vi "Channels data blend.vi"(8 "error in (no error)":errorcluster, 10 "GREEN":T1, 11 "RED":T1) -> (0 "error out":errorcluster, 3 "Image Out":T1)   [LabVIEW 2020]
uses:
  <vilib>/vision/Image Controls.llb/IMAQ Image.ctl
  <vilib>/vision/NI_Vision_Development_Module.lvlib
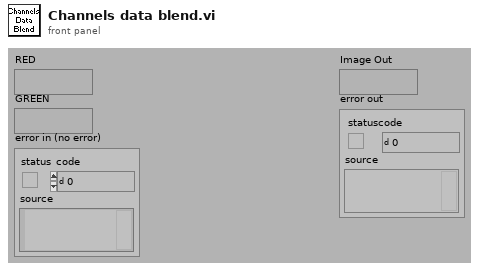
[diagram p1: front panel]
types:
  T1 = typedef "IMAQ Image.ctl" = refnum<image>
  T2 = typedef "Image Type" = u32
  T3 = cluster{"Red or Hue value":u8, "Green or Sat value":u8, "Blue or Luma or Val or Inten value":u8}
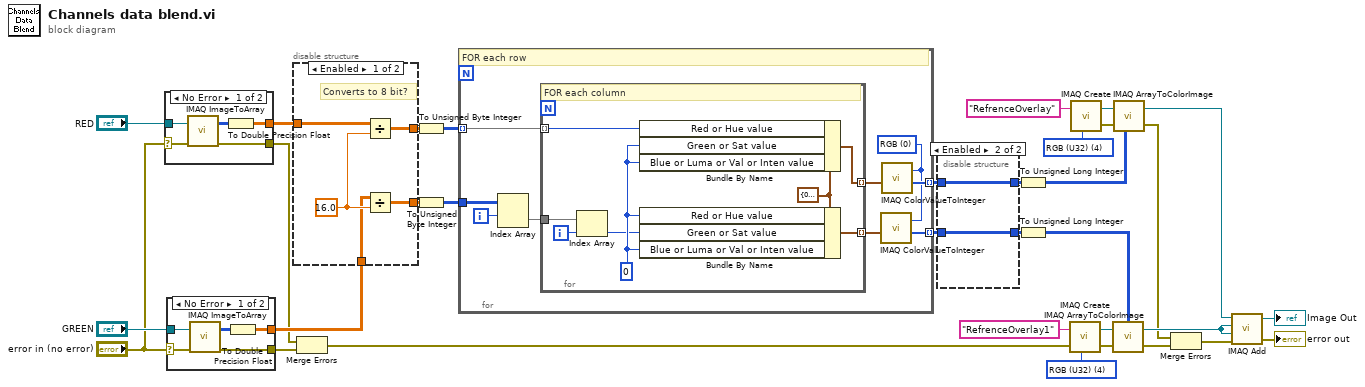
[diagram p0: block diagram]
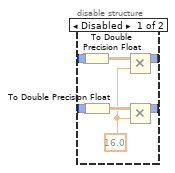
[diagram p2: hidden frame]
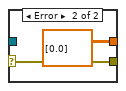
[diagram p4: hidden frame]
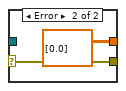
[diagram p5: hidden frame]
diagram:
  w28 = T2 4 items=["Grayscale (U8)", "Grayscale (I16)", "Grayscale (SGL)", "Complex (CSG)", "RGB (U32)", "HSL (U32)", "RGB (U64)", "Grayscale (U16)"] ("Image Type")
  w33 = T2 4 items=["Grayscale (U8)", "Grayscale (I16)", "Grayscale (SGL)", "Complex (CSG)", "RGB (U32)", "HSL (U32)", "RGB (U64)", "Grayscale (U16)"] ("Image Type")
  n1 = case shown="No Error" "error in (no error)" {
    selector: "error in (no error)" -> [w36 w39]
    tunnel: [w34 dbl[][] [[0.0]] ("Image Pixels (I16)")] -> w11
    tunnel: "RED" -> [w38 _]
    tunnel: [w37 w39] -> w9
    frame No Error {
      n2 = call "IMAQ ImageToArray"("error in (no error)"=w36, "Image"=w38) -> ("error out"=w37:errorcluster, "Image Pixels (I16)"=w35:i16[][])  [unwired: 2 in, 3 out]
      n3 = To Double Precision Float(number=w35) -> (double precision float=w34:dbl[][])
    }
    frame Error {
    }
  }
  n4 = case shown="No Error" "error in (no error)" {
    selector: "error in (no error)" -> [w43 w46]
    tunnel: [w41 dbl[][] [[0.0]] ("Image Pixels (I16)")] -> w13
    tunnel: "GREEN" -> [w45 _]
    tunnel: [w44 w46] -> w7
    frame No Error {
      n5 = call "IMAQ ImageToArray"("error in (no error)"=w43, "Image"=w45) -> ("error out"=w44:errorcluster, "Image Pixels (I16)"=w42:i16[][])  [unwired: 2 in, 3 out]
      n6 = To Double Precision Float(number=w42) -> (double precision float=w41:dbl[][])
    }
    frame Error {
    }
  }
  n7 = disable-structure shown="Enabled" {
    disable-tunnel: [w52 w54] -> w21
    disable-tunnel: [w51 w53] -> w19
    disable-tunnel: w13 -> [w49 w53]
    disable-tunnel: w11 -> [w48 w54]
    frame Enabled {
      w50 = 16.0
      # "Converts to 8 bit?"
      n8 = Divide(x=w48, y=w50) -> (x/y=w52:dbl[][])
      n9 = Divide(x=w49, y=w50) -> (x/y=w51:dbl[][])
    }
    frame Disabled {
    }
  }
  n10 = Merge Errors(w9, w7) -> (w8:errorcluster)
  n11 = To Unsigned Byte Integer(number=w21) -> (unsigned 8bit integer=w20:u8[][])
  n12 = To Unsigned Byte Integer(number=w19) -> (unsigned 8bit integer=w18:u8[][])
  n13 = for {
    tunnel: w20 -> [w63] mode=indexing
    tunnel: w18 -> [w58]
    tunnel: [w59] -> w5 mode=indexing
    tunnel: [w61] -> w2 mode=indexing
    i -> [w56]
    w55 = u16 0 items=["RGB", "HSL", "HSV", "HSI"] ("Color Mode")
    # "FOR each row"
    n14 = Index Array(array=w58, index (row)=w56) -> (element=w57:u8[])  [unwired: 1 in]
    n15 = for {
      tunnel: w63 -> [w71] mode=indexing
      tunnel: w57 -> [w66]
      tunnel: [w69] -> w62 mode=indexing
      tunnel: [w68] -> w60 mode=indexing
      i -> [w65]
      w67 = T3 {"Red or Hue value"=0, "Green or Sat value"=0, "Blue or Luma or Val or Inten value"=0} ("Color Value")
      w70 = u8 0
      # "FOR each column"
      n16 = Index Array(array=w66, index=w65) -> (element=w64:u8)
      n17 = Bundle By Name(cluster=w67, "Red or Hue value"=w71, "Green or Sat value"=w70, "Blue or Luma or Val or Inten value"=w70) -> (w68:T3)
      n18 = Bundle By Name(cluster=w67, "Red or Hue value"=w70, "Green or Sat value"=w64, "Blue or Luma or Val or Inten value"=w70) -> (w69:T3)
    }
    n19 = call "IMAQ ColorValueToInteger"("1D Color value array"=w62, "Color Mode"=w55) -> ("1D U32 array"=w61:u32[])  [unwired: 3 in, 3 out]
    n20 = call "IMAQ ColorValueToInteger"("1D Color value array"=w60, "Color Mode"=w55) -> ("1D U32 array"=w59:u32[])  [unwired: 3 in, 3 out]
  }
  n21 = disable-structure shown="Enabled" {
    disable-tunnel: [w78 w80] -> w6
    disable-tunnel: w5 -> [w77 w80]
    disable-tunnel: [w74 w79] -> w3
    disable-tunnel: w2 -> [w73 w79]
    frame Disabled {
      w72 = 16.0
      n22 = To Double Precision Float(number=w77) -> (double precision float=w76:dbl[][])
      n23 = To Double Precision Float(number=w73) -> (double precision float=w75:dbl[][])
      n24 = Multiply(x=w76, y=w72) -> (x*y=w78:dbl[][])
      n25 = Multiply(x=w75, y=w72) -> (x*y=w74:dbl[][])
    }
    frame Enabled {
    }
  }
  n26 = To Unsigned Long Integer(number=w6) -> (unsigned 32bit integer=w4:u32[][])
  n27 = To Unsigned Long Integer(number=w3) -> (unsigned 32bit integer=w1:u32[][])
  n28 = call "IMAQ Create"("Image Name"="RefrenceOverlay1", "Image Type"=w28, "error in (no error)"=w8) -> ("New Image"=w27:T1, "error out"=w26:errorcluster)  [unwired: 2 in]
  n29 = call "IMAQ Create"("Image Name"="RefrenceOverlay", "Image Type"=w33) -> ("New Image"=w32:T1, "error out"=w31:errorcluster)  [unwired: 3 in]
  n30 = call "IMAQ ArrayToColorImage"("Image Pixels (U32)"=w1, "Image"=w27, "error in (no error)"=w26) -> ("Image Out"=w24:T1, "error out"=w16:errorcluster)  [unwired: 2 in]
  n31 = call "IMAQ ArrayToColorImage"("Image Pixels (U32)"=w4, "Image"=w32, "error in (no error)"=w31) -> ("Image Out"=w23:T1, "error out"=w17:errorcluster)  [unwired: 2 in]
  n32 = Merge Errors(w17, w16) -> (w15:errorcluster)
  n33 = call "IMAQ Add"("Image Src A"=w23, "Image Dst"=w24, "Image Src B"=w24, "error in (no error)"=w15) -> ("Image Dst Out"=→"Image Out":T1, "error out"=→"error out":errorcluster)  [unwired: 3 in]
